vi "updateCommandStringDL.vi"(8 "error in (no error)":errorcluster, 10 "Command U8 Array":u8[](array[numeric]), 11 "MiddlewareSALThisComponent in":refnum<class "MiddlewareSALThisComponent.lvclass">) -> (0 "error out":errorcluster, 2 "Cmd str":string, 3 "MiddlewareSALThisComponent out":refnum<class "MiddlewareSALThisComponent.lvclass">)   [LabVIEW 2016, in "MiddlewareSALThisComponent.lvclass"]
uses:
  MiddlewareSALThisComponent.lvclass
  ComponentTemplateCore/ComponentModel/ComponentModel/Command/Command.lvclass
  Commands/Start/start.lvclass
  ts_sallv_sedspectrometer/SALLV_sedSpectrometer.lvlib
  Commands/CaptureSpectImage/captureSpectImage.lvclass
  home/harini/tcs/ts_sedspectrometer/CommandThisComponent/CommandThisComponent.lvclass
  home/harini/tcs/ts_sedspectrometer/ComponentTemplateCore/ComponentModel/ComponentModel/Command/Command.lvclass
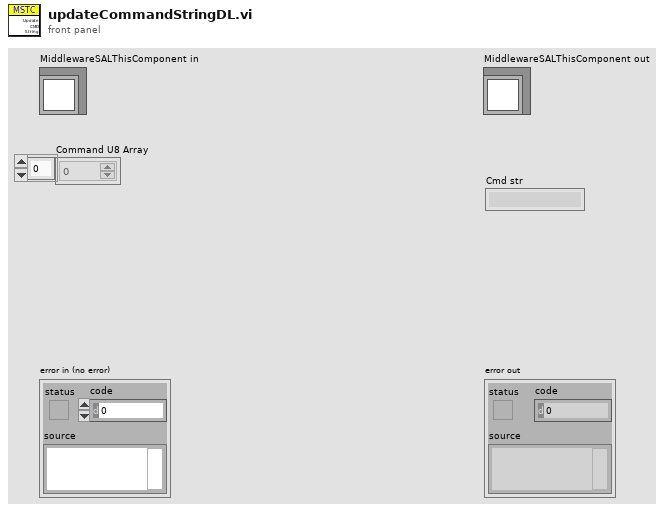
[diagram p1: front panel]
types:
  T1 = typedef "SEDSpectrometerTypedefs.lvlib/CommandValue.ctl" = enum16{"clearError", "disable", "enable", "exit", "GoToStandby", "OnHeartbeat", "OnIncomingMessagingError", "OnInterrupt", "start", "captureSpectImage", "setSpectTempSetpoint", "stopImageCapture"}
  T2 = typedef "SALLV_sedSpectrometer.lvlib/command_start.ctl" = cluster{"settingsToApply":string}
  T3 = typedef "SALLV_sedSpectrometer.lvlib/command_captureSpectImage.ctl" = cluster{"integrationTime":sgl, "imageType":string, "lamp":string}
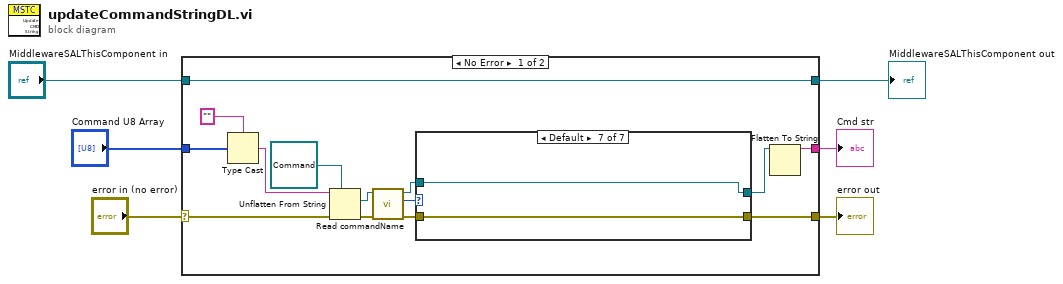
[diagram p0: block diagram]
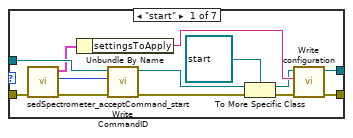
[diagram p2: hidden frame]
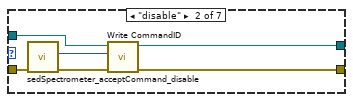
[diagram p3: hidden frame]
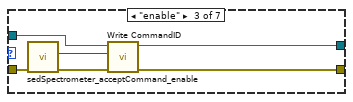
[diagram p4: hidden frame]
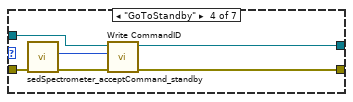
[diagram p5: hidden frame]
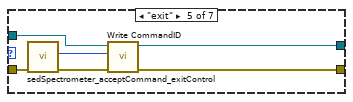
[diagram p6: hidden frame]
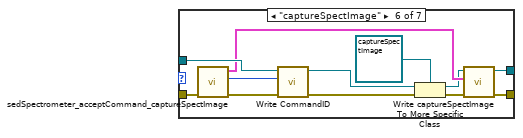
[diagram p7: hidden frame]
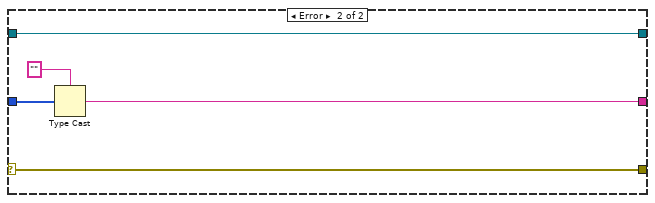
[diagram p8: hidden frame]
diagram:
  n1 = case shown="No Error" "error in (no error)" {
    selector: "error in (no error)" -> [w16 w76]
    tunnel: [w11 w76] -> w5
    tunnel: [w7 w75] -> w3
    tunnel: "MiddlewareSALThisComponent in" -> [w7 w75]
    tunnel: "Command U8 Array" -> [w17 w74]
    tunnel: [w8 w72] -> w1
    frame No Error {
      n2 = Type Cast(type="", x=w17) -> (*(type *) &x=w18:string)
      n3 = Unflatten From String(type=refnum<class "Command.lvclass"> refnum ("Command.lvclass"), binary string=w18, error in (no error)=w16) -> (value=w14:refnum<class "Command.lvclass">, error out=w15:errorcluster)  [unwired: 2 in, 1 out]
      n4 = call-dynamic "Read commandName.vi"("error in (no error)"=w15, "Command in"=w14) -> ("error out"=w13:errorcluster, "CommandValue"=w10:T1, "Command out"=w12:refnum<class "Command.lvclass">)  [unwired: 7 in]
      n5 = case shown="Default" w10 {
        tunnel: w13 -> [w33 w39 w42 w46 w52 w69 w71]
        tunnel: [w26 w34 w45 w50 w55 w59 w71] -> w11
        tunnel: w12 -> [w32 w36 w43 w51 w57 w64 w70]
        tunnel: [w22 w35 w44 w49 w56 w58 w70] -> w9
        frame "start" {
          n6 = call "sedSpectrometer_acceptCommand_start.vi"("error in (no error)"=w33) -> ("error out"=w30:errorcluster, "function return"=w31:i32, "command_start_Ctl out"=w25:T2)  [unwired: 8 in]
          n7 = Unbundle By Name(w25) -> ("settingsToApply"=w24:string)
          n8 = call-dynamic "Write CommandID.vi"("error in (no error)"=w30, "CommandID"=w31, "Command in"=w32) -> ("error out"=w29:errorcluster, "Command out"=w21:refnum<class "Command.lvclass">)  [unwired: 7 in]
          n9 = To More Specific Class(target class=refnum<class "start.lvclass"> refnum ("Commands.lvlib:start.lvclass"), reference=w21, error in=w29) -> (specific class reference=w23:refnum<class "start.lvclass">, error out=w27:errorcluster)
          n10 = call-dynamic "Write configuration.vi"("error in (no error)"=w27, "configuration"=w24, "Start in"=w23) -> ("error out"=w26:errorcluster, "Start out"=w22:refnum<class "start.lvclass">)  [unwired: 7 in]
        }
        frame "disable" {
          n11 = call "sedSpectrometer_acceptCommand_disable.vi"("error in (no error)"=w39) -> ("error out"=w38:errorcluster, "function return"=w37:i32)  [unwired: 8 in, 1 out]
          n12 = call-dynamic "Write CommandID.vi"("error in (no error)"=w38, "CommandID"=w37, "Command in"=w36) -> ("error out"=w34:errorcluster, "Command out"=w35:refnum<class "Command.lvclass">)  [unwired: 7 in]
        }
        frame "enable" {
          n13 = call "sedSpectrometer_acceptCommand_enable.vi"("error in (no error)"=w42) -> ("error out"=w41:errorcluster, "function return"=w40:i32)  [unwired: 8 in, 1 out]
          n14 = call-dynamic "Write CommandID.vi"("error in (no error)"=w41, "CommandID"=w40, "Command in"=w43) -> ("error out"=w45:errorcluster, "Command out"=w44:refnum<class "Command.lvclass">)  [unwired: 7 in]
        }
        frame "GoToStandby" {
          n15 = call "sedSpectrometer_acceptCommand_standby.vi"("error in (no error)"=w46) -> ("error out"=w48:errorcluster, "function return"=w47:i32)  [unwired: 8 in, 1 out]
          n16 = call-dynamic "Write CommandID.vi"("error in (no error)"=w48, "CommandID"=w47, "Command in"=w51) -> ("error out"=w50:errorcluster, "Command out"=w49:refnum<class "Command.lvclass">)  [unwired: 7 in]
        }
        frame "exit" {
          n17 = call "sedSpectrometer_acceptCommand_exitControl.vi"("error in (no error)"=w52) -> ("error out"=w54:errorcluster, "function return"=w53:i32)  [unwired: 8 in, 1 out]
          n18 = call-dynamic "Write CommandID.vi"("error in (no error)"=w54, "CommandID"=w53, "Command in"=w57) -> ("error out"=w55:errorcluster, "Command out"=w56:refnum<class "Command.lvclass">)  [unwired: 7 in]
        }
        frame "captureSpectImage" {
          n19 = call "sedSpectrometer_acceptCommand_captureSpectImage.vi"("error in (no error)"=w69) -> ("error out"=w66:errorcluster, "function return"=w65:i32, "command_captureSpectImage_Ctl out"=w62:T3)  [unwired: 8 in]
          n20 = call-dynamic "Write CommandID.vi"("error in (no error)"=w66, "CommandID"=w65, "Command in"=w64) -> ("error out"=w67:errorcluster, "Command out"=w68:refnum<class "Command.lvclass">)  [unwired: 7 in]
          n21 = To More Specific Class(target class=refnum<class "captureSpectImage.lvclass"> refnum ("Commands.lvlib:CaptureSpectImage.lvclass"), reference=w68, error in=w67) -> (specific class reference=w61:refnum<class "captureSpectImage.lvclass">, error out=w60:errorcluster)
          n22 = call-dynamic "Write captureSpectImage.vi"("error in (no error)"=w60, "command_captureSpectImage"=w62, "captureSpectImage in"=w61) -> ("error out"=w59:errorcluster, "captureSpectImage out"=w58:refnum<class "captureSpectImage.lvclass">)  [unwired: 7 in]
        }
        frame Default {
        }
      }
      n23 = Flatten To String(anything=w9) -> (data string=w8:string)  [unwired: 3 in, 2 out]
    }
    frame Error {
      n24 = Type Cast(type="", x=w74) -> (*(type *) &x=w72:string)
    }
  }
  "error out" <- w5
  "MiddlewareSALThisComponent out" <- w3
  "Cmd str" <- w1
